vi "Host 25035.vi"() -> ()   [LabVIEW 2018]
uses:
  <instrlib>/niDCPower/nidcpower.llb/niDCPower Measurement Type.ctl
panel:
  in  "2.1_selcur":dbl=0.3 caption="current limit" format="%_6p"
  out "2.1":i32
  out "2.1":bool
  in  "2.0_selcur":dbl=0.3 caption="current limit" format="%_6p"
  out "2.0":i32
  out "2.0":bool
  in  "2.1, V":dbl=5.0 caption="voltage level" format="%_6p"
  in  "2.1_curlim, A":dbl=0.5 caption="current limit" format="%_6p"
  out "2.1_cur, A":dbl caption="measurement" format="%_6g"
  out "2.1 Chart":dbl(graph)=-0.007994936055928669 caption="Waveform Chart 5"
  in  "Период опроса, мс":u32=1
  out "2.0_cur, A":dbl caption="measurement" format="%_6g"
  out "2.0 Chart":dbl(graph)=0.03234747481509968 caption="Waveform Chart 5"
  in  "2.0, V":dbl=5.0 caption="voltage level" format="%_6p"
  in  "2.0_curlim, A":dbl=0.5 caption="current limit" format="%_6p"
  in  "2.0/2.1":refnum<k15>="PXI1Slot4" caption="instrument handle"
  in  "1.1_selcur":dbl=0.3 caption="current limit" format="%_6p"
  out "1.1":i32
  out "1.1":bool
  out "1.1_cur, A":dbl caption="measurement" format="%_6g"
  out "1.1 Chart":dbl(graph)=-0.000235222149982668
  in  "1.1, V":dbl=5.0 caption="voltage level" format="%_6p"
  in  "1.1_curlim, A":dbl=0.5 caption="current limit" format="%_6p"
  in  "Стоп":bool
  in  "Питание":bool
  in  "SEL_T, мс":u32=100
  in  "SIM_SEL":bool
  out "SEL":bool
  in  "0.0_selcur":dbl=0.3 caption="current limit" format="%_6p"
  in  "0.1_selcur":dbl=0.3 caption="current limit" format="%_6p"
  in  "1.0_selcur":dbl=0.3 caption="current limit" format="%_6p"
  out "0.0":i32
  out "0.0":bool
  out "0.1":i32
  out "0.1":bool
  out "1.0":i32
  out "1.0":bool
  in  "0.0, V":dbl=5.0 caption="voltage level" format="%_6p"
  in  "0.0_curlim, A":dbl=0.5 caption="current limit" format="%_6p"
  in  "0.1_curlim, A":dbl=0.5 caption="current limit" format="%_6p"
  out "0.0_cur, A":dbl caption="measurement" format="%_6g"
  out "0.1_cur, A":dbl caption="measurement" format="%_6g"
  in  "0.1, V":dbl=5.0 caption="voltage level" format="%_6p"
  in  "1.0, V":dbl=5.0 caption="voltage level" format="%_6p"
  in  "1.0_curlim, A":dbl=0.5 caption="current limit" format="%_6p"
  out "1.0_cur, A":dbl caption="measurement" format="%_6g"
  out "0.1 Chart":dbl(graph)=-0.0025072983641264367
  out "1.0 Chart":dbl(graph)=-0.0403673797130392
  out "0.0 Chart":dbl(graph)=0.17110122624002952 caption="Waveform Chart 5"
  in  "0.0/0.1":refnum<k15>="PXI1Slot2" caption="instrument handle"
  in  "1.0/1.1":refnum<k15>="PXI1Slot3" caption="instrument handle"
  in  "SEL":path=path "C:/LabView_PRJ/25_035_ИКИ РАН/SEL"
  out "Номер образца":string="0"
  # "Для ТЗЧ:\n0.0 - питание ПЛИС\n1.0 - питание матрицы"
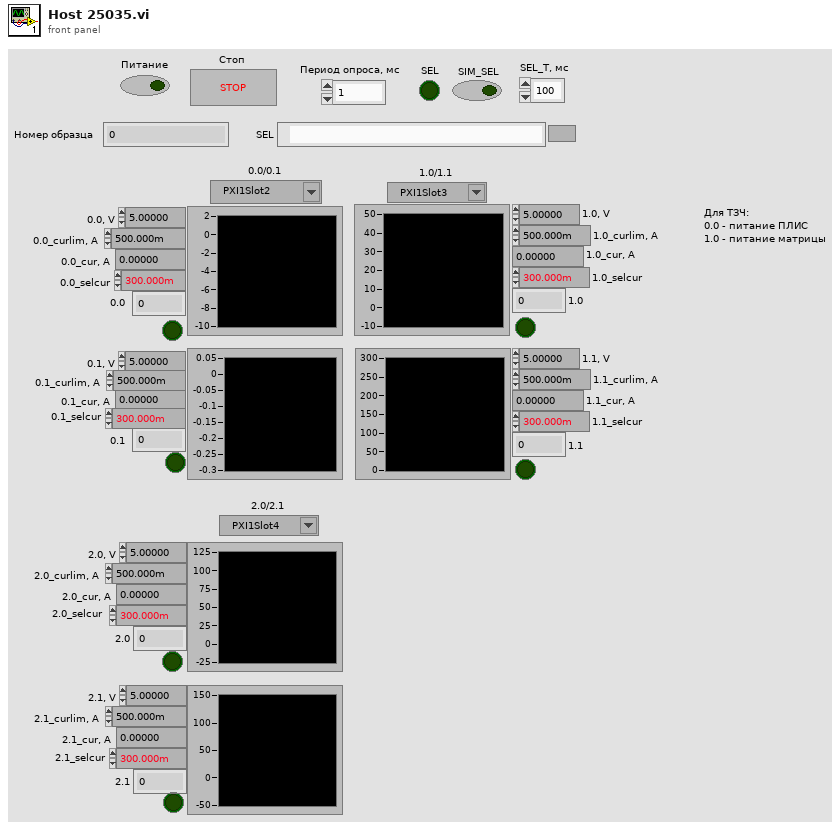
[diagram p1: front panel]
types:
  T1 = enum16{"open", "replace", "create", "open or create", "replace or create", "replace or create with confirmation"}
  T2 = typedef "niDCPower Measurement Type.ctl" = i32
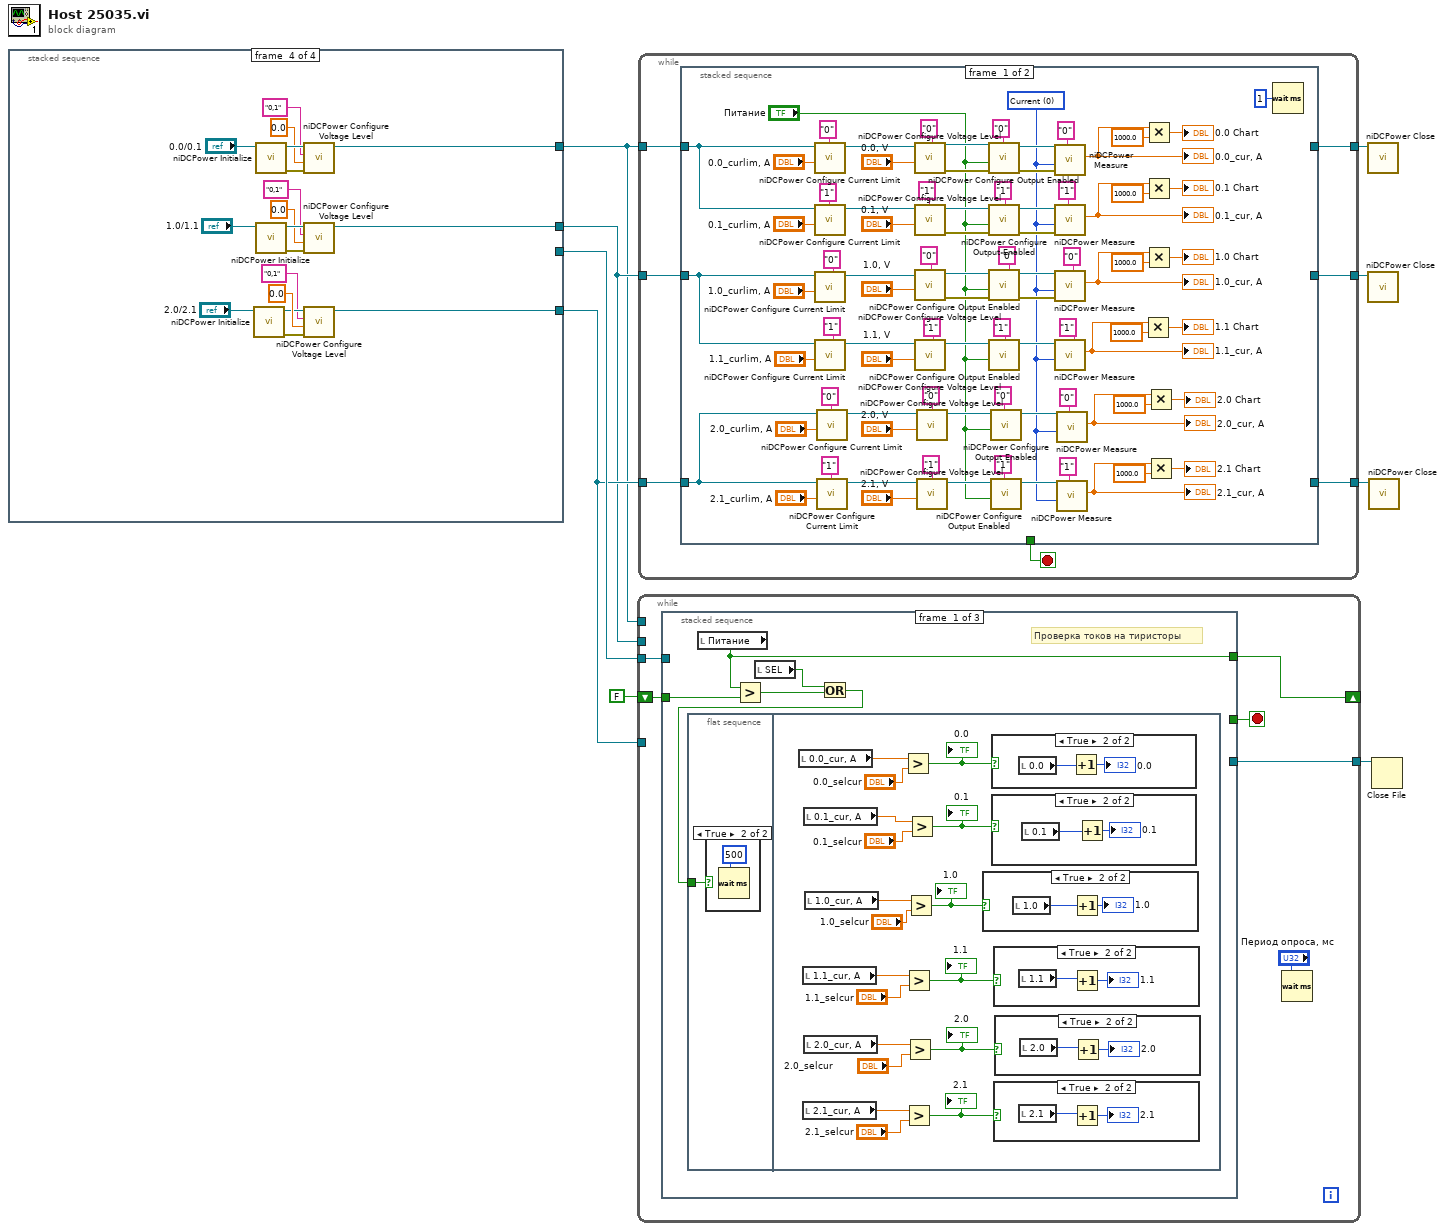
[diagram p0: block diagram]
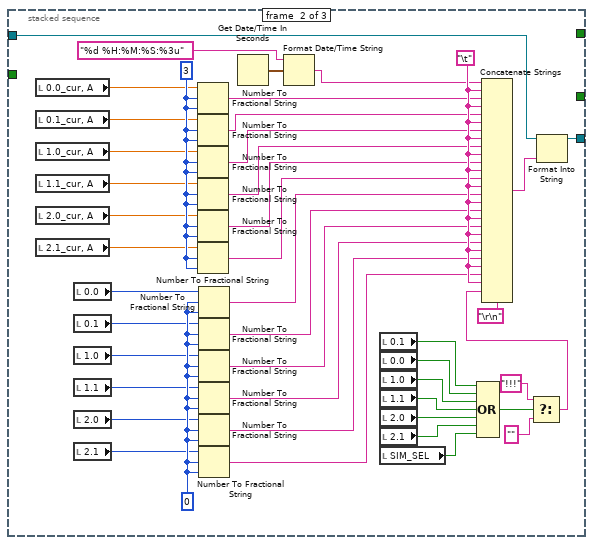
[diagram p9: hidden frame]
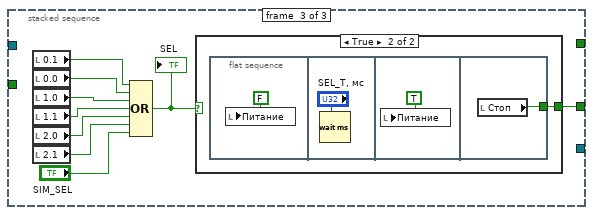
[diagram p10: hidden frame]
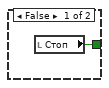
[diagram p11: hidden frame]
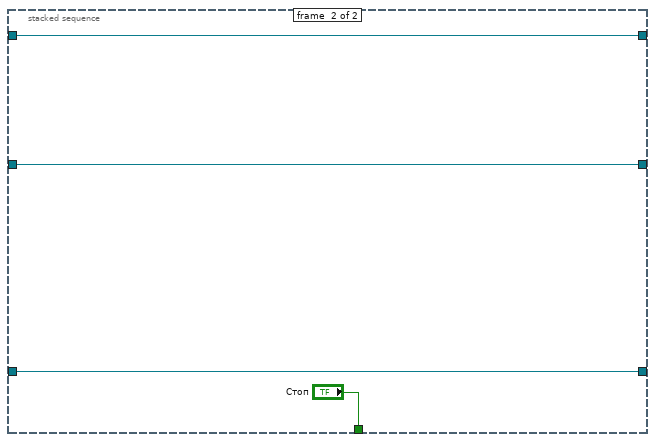
[diagram p12: hidden frame]
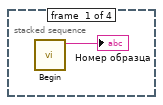
[diagram p13: hidden frame]
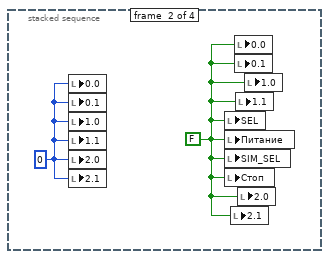
[diagram p14: hidden frame]
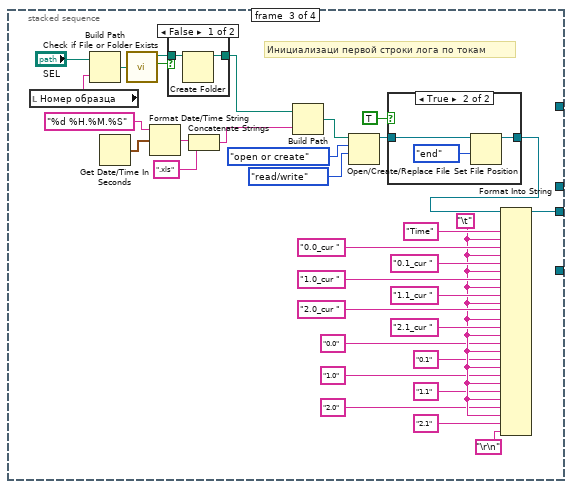
[diagram p15: hidden frame]
diagram:
  n1 = stacked-sequence {
    tunnel: [_ _ _ w60] -> w5
    tunnel: [_ _ _ w59] -> w4
    tunnel: [_ _ w29 _] -> w8
    tunnel: [_ _ _ w53] -> w6
    frame #0 {
      n2 = call "Begin.vi"() -> ("Номер образца 2"=→"Номер образца":string)  [unwired: 11 in]
    }
    frame #1 {
      w12 = 0
      w11 = FALSE
      n3 = local write "0.0"(w12) -> ()
      n4 = local write "0.1"(w12) -> ()
      n5 = local write "1.0"(w12) -> ()
      n6 = local write "1.1"(w12) -> ()
      n7 = local write "2.0"(w12) -> ()
      n8 = local write "2.1"(w12) -> ()
      n9 = local write "SEL"(w11) -> ()
      n10 = local write "Питание"(w11) -> ()
      n11 = local write "SIM_SEL"(w11) -> ()
      n12 = local write "Стоп"(w11) -> ()
      n13 = local write "2.1"(w11) -> ()
      n14 = local write "0.0"(w11) -> ()
      n15 = local write "0.1"(w11) -> ()
      n16 = local write "1.1"(w11) -> ()
      n17 = local write "2.0"(w11) -> ()
      n18 = local write "1.0"(w11) -> ()
    }
    frame #2 {
      w20 = "\t"
      # "Инициализаци первой строки лога по токам"
      n19 = local read "Номер образца"() -> (w41:string)
      n20 = Build Path(base path="SEL", name or relative path=w41) -> (appended path=w43:path)
      n21 = Get Date/Time In Seconds() -> (seconds since 1Jan1904=w36:timestamp)
      n22 = call <vilib>:"Check if File or Folder Exists.vi"("path"=w43) -> ("file or folder exists?"=w44:bool, "dup path"=w45:path)  [unwired: 8 in, 1 out]
      n23 = Format Date/Time String(time format string (%c)="%d %H.%M.%S", seconds (now)=w36) -> (date/time string=w33:string)  [unwired: 1 in]
      n24 = case shown="False" w44 {
        tunnel: w45 -> [w51 w52]
        tunnel: [w50 w52] -> w28
        frame False {
          n25 = Create Folder(path (use dialog)=w51) -> (created path=w50:path)  [unwired: 2 in, 2 out]
        }
        frame True {
        }
      }
      n26 = Concatenate Strings(w33, ".xls" ("string")) -> (w31:string)
      n27 = Build Path(base path=w28, name or relative path=w31) -> (appended path=w34:path)
      n28 = Open/Create/Replace File(file path (use dialog)=w34, operation (0:open)=T1."open or create", access (0:read/write)=enum16{"read/write", "read-only", "write-only"}."read/write") -> (refnum out=w37:refnum<file>)  [unwired: 3 in, 2 out]
      n29 = case shown="True" TRUE {
        tunnel: w37 -> [w46 w49]
        tunnel: [w46 w47] -> w30
        frame False {
        }
        frame True {
          n30 = Set File Position(refnum=w49, from (0:start)=enum16{"start", "end", "current"}."end") -> (refnum out=w47:refnum<file>)  [unwired: 2 in, 1 out]
        }
      }
      n31 = Format Into String(initial string=w30, "Time" ("input 1"), w20, "0.0_cur " ("input 1"), w20, "0.1_cur " ("input 1"), w20, "1.0_cur " ("input 1"), w20, "1.1_cur " ("input 1"), w20, "2.0_cur " ("input 1"), w20, "2.1_cur " ("input 1"), w20, "0.0" ("input 1"), w20, "0.1" ("input 1"), w20, "1.0" ("input 1"), w20, "1.1" ("input 1"), w20, "2.0" ("input 1"), w20, "2.1" ("input 1"), "\r\n") -> (resulting string=w29:refnum<file>)  [unwired: 2 in, 1 out]
    }
    frame #3 {
      n32 = call <instrlib>:"niDCPower Initialize.vi"("resource name"="2.0/2.1") -> ("error out"=w56:errorcluster, "instrument handle out"=w55:refnum<k15>)  [unwired: 3 in, 6 out]
      n33 = call <instrlib>:"niDCPower Initialize.vi"("resource name"="0.0/0.1") -> ("error out"=w67:errorcluster, "instrument handle out"=w69:refnum<k15>)  [unwired: 3 in, 6 out]
      n34 = call <instrlib>:"niDCPower Initialize.vi"("resource name"="1.0/1.1") -> ("error out"=w68:errorcluster, "instrument handle out"=w70:refnum<k15>)  [unwired: 3 in, 6 out]
      n35 = call <instrlib>:"niDCPower Configure Voltage Level.vi"("error in (no error)"=w67, "voltage level"=0.0, "channel name"="0,1", "instrument handle"=w69) -> ("instrument handle out"=w59:refnum<k15>)  [unwired: 6 in, 1 out]
      n36 = call <instrlib>:"niDCPower Configure Voltage Level.vi"("error in (no error)"=w68, "voltage level"=0.0, "channel name"="0,1", "instrument handle"=w70) -> ("instrument handle out"=w60:refnum<k15>)  [unwired: 6 in, 1 out]
      n37 = call <instrlib>:"niDCPower Configure Voltage Level.vi"("error in (no error)"=w56, "voltage level"=0.0, "channel name"="0,1", "instrument handle"=w55) -> ("instrument handle out"=w53:refnum<k15>)  [unwired: 6 in, 1 out]
    }
  }
  n38 = while {
    shift-right: [w76] -> _
    shift-left: FALSE -> [w75]
    tunnel: w8 -> [w74]
    tunnel: [w72] -> w7
    tunnel: w6 -> [_]
    tunnel: w5 -> [_]
    tunnel: w4 -> [_]
    stop <- w73 stop-if-true
    n39 = stacked-sequence {
      tunnel: [w80 _ _] -> w76
      tunnel: w75 -> [w81 _ _]
      tunnel: w74 -> [_ w153 _]
      tunnel: [_ _ w167] -> w73
      tunnel: [_ w152 _] -> w72
      frame #0 {
        # "Проверка токов на тиристоры"
        n40 = flat-sequence {
          tunnel: w77 -> [w82]
          frame #0 {
            n41 = case shown="True" w82 {
              frame False {
              }
              frame True {
                n42 = Wait (ms)(milliseconds to wait=u32 500) -> ()  [unwired: 1 out]
              }
            }
          }
          frame #1 {
            n43 = local read "0.0_cur, A"() -> (w95:dbl)
            n44 = local read "1.1_cur, A"() -> (w92:dbl)
            n45 = local read "2.1_cur, A"() -> (w86:dbl)
            n46 = local read "0.1_cur, A"() -> (w94:dbl)
            n47 = local read "2.0_cur, A"() -> (w87:dbl)
            n48 = local read "1.0_cur, A"() -> (w93:dbl)
            n49 = Greater?(x=w95, y="0.0_selcur") -> (0:w100:bool)
            "0.0" <- w100
            n50 = Greater?(x=w92, y="1.1_selcur") -> (0:w91:bool)
            "1.1" <- w91
            n51 = Greater?(x=w86, y="2.1_selcur") -> (0:w85:bool)
            "2.1" <- w85
            n52 = Greater?(x=w87, y="2.0_selcur") -> (0:w88:bool)
            "2.0" <- w88
            n53 = Greater?(x=w93, y="1.0_selcur") -> (0:w96:bool)
            "1.0" <- w96
            n54 = Greater?(x=w94, y="0.1_selcur") -> (0:w98:bool)
            "0.1" <- w98
            n55 = case shown="True" w96 {
              frame False {
              }
              frame True {
                n56 = local read "1.0"() -> (w109:i32)
                n57 = Increment(x=w109) -> (x+1=→"1.0":i32)
              }
            }
            n58 = case shown="True" w100 {
              frame False {
              }
              frame True {
                n59 = local read "0.0"() -> (w113:i32)
                n60 = Increment(x=w113) -> (x+1=→"0.0":i32)
              }
            }
            n61 = case shown="True" w98 {
              frame False {
              }
              frame True {
                n62 = local read "0.1"() -> (w110:i32)
                n63 = Increment(x=w110) -> (x+1=→"0.1":i32)
              }
            }
            n64 = case shown="True" w91 {
              frame False {
              }
              frame True {
                n65 = local read "1.1"() -> (w107:i32)
                n66 = Increment(x=w107) -> (x+1=→"1.1":i32)
              }
            }
            n67 = case shown="True" w85 {
              frame False {
              }
              frame True {
                n68 = local read "2.1"() -> (w103:i32)
                n69 = Increment(x=w103) -> (x+1=→"2.1":i32)
              }
            }
            n70 = case shown="True" w88 {
              frame False {
              }
              frame True {
                n71 = local read "2.0"() -> (w105:i32)
                n72 = Increment(x=w105) -> (x+1=→"2.0":i32)
              }
            }
          }
        }
        n73 = local read "Питание"() -> (w80:bool)
        n74 = Greater?(x=w80, y=w81) -> (0:w79:bool)
        n75 = local read "SEL"() -> (w78:bool)
        n76 = Or(x=w78, y=w79) -> (x .or. y?=w77:bool)
      }
      frame #1 {
        w150 = i16 0 ("width (-)")
        w151 = i16 3 ("width (-)")
        w149 = "\t"
        n77 = local read "0.0_cur, A"() -> (w148:dbl)
        n78 = local read "0.1_cur, A"() -> (w147:dbl)
        n79 = local read "1.0_cur, A"() -> (w146:dbl)
        n80 = local read "1.1_cur, A"() -> (w145:dbl)
        n81 = local read "2.0_cur, A"() -> (w144:dbl)
        n82 = local read "2.1_cur, A"() -> (w143:dbl)
        n83 = local read "0.0"() -> (w142:i32)
        n84 = local read "0.1"() -> (w141:i32)
        n85 = local read "1.0"() -> (w140:i32)
        n86 = local read "1.1"() -> (w139:i32)
        n87 = local read "2.0"() -> (w138:i32)
        n88 = local read "2.1"() -> (w137:i32)
        n89 = Number To Fractional String(number=w148, width (-)=w151, precision (6)=w151) -> (F-format string=w135:string)  [unwired: 1 in]
        n90 = Number To Fractional String(number=w147, width (-)=w151, precision (6)=w151) -> (F-format string=w134:string)  [unwired: 1 in]
        n91 = Number To Fractional String(number=w146, width (-)=w151, precision (6)=w151) -> (F-format string=w133:string)  [unwired: 1 in]
        n92 = Number To Fractional String(number=w145, width (-)=w151, precision (6)=w151) -> (F-format string=w132:string)  [unwired: 1 in]
        n93 = Number To Fractional String(number=w144, width (-)=w151, precision (6)=w151) -> (F-format string=w131:string)  [unwired: 1 in]
        n94 = Number To Fractional String(number=w143, width (-)=w151, precision (6)=w151) -> (F-format string=w130:string)  [unwired: 1 in]
        n95 = Number To Fractional String(number=w142, width (-)=w150, precision (6)=w150) -> (F-format string=w129:string)  [unwired: 1 in]
        n96 = Number To Fractional String(number=w141, width (-)=w150, precision (6)=w150) -> (F-format string=w128:string)  [unwired: 1 in]
        n97 = Number To Fractional String(number=w140, width (-)=w150, precision (6)=w150) -> (F-format string=w127:string)  [unwired: 1 in]
        n98 = Number To Fractional String(number=w139, width (-)=w150, precision (6)=w150) -> (F-format string=w126:string)  [unwired: 1 in]
        n99 = Number To Fractional String(number=w138, width (-)=w150, precision (6)=w150) -> (F-format string=w125:string)  [unwired: 1 in]
        n100 = Number To Fractional String(number=w137, width (-)=w150, precision (6)=w150) -> (F-format string=w124:string)  [unwired: 1 in]
        n101 = Get Date/Time In Seconds() -> (seconds since 1Jan1904=w158:timestamp)
        n102 = Format Date/Time String(time format string (%c)="%d %H:%M:%S:%3u", seconds (now)=w158) -> (date/time string=w136:string)  [unwired: 1 in]
        n103 = local read "0.1"() -> (w121:bool)
        n104 = local read "0.0"() -> (w120:bool)
        n105 = local read "1.0"() -> (w119:bool)
        n106 = local read "1.1"() -> (w118:bool)
        n107 = local read "2.0"() -> (w117:bool)
        n108 = local read "2.1"() -> (w116:bool)
        n109 = local read "SIM_SEL"() -> (w115:bool)
        n110 = Compound Arithmetic op=OR(w121, w120, w119, w118, w117, w116, w115) -> (w114:bool)
        n111 = Select(t="!!!", s=w114, f="") -> (s? t:f=w123:string)
        n112 = Concatenate Strings(w136, w149, w135, w149, w134, w149, w133, w149, w132, w149, w131, w149, w130, w149, w129, w149, w128, w149, w127, w149, w126, w149, w125, w149, w124, w149, w123, "\r\n") -> (w157:string)
        n113 = Format Into String(initial string=w153, w157) -> (resulting string=w152:refnum<file>)  [unwired: 2 in, 1 out]
      }
      frame #2 {
        n114 = local read "0.1"() -> (w166:bool)
        n115 = local read "0.0"() -> (w164:bool)
        n116 = local read "1.0"() -> (w163:bool)
        n117 = local read "1.1"() -> (w162:bool)
        n118 = local read "2.0"() -> (w161:bool)
        n119 = local read "2.1"() -> (w160:bool)
        n120 = Compound Arithmetic op=OR(w166, w164, w163, w162, w161, w160, "SIM_SEL") -> (w165:bool)
        "SEL" <- w165
        n121 = case shown="True" w165 {
          tunnel: [w168 w169] -> w167
          frame False {
            n122 = local read "Стоп"() -> (w168:bool)
          }
          frame True {
            n123 = flat-sequence {
              tunnel: [w173] -> w169
              frame #0 {
                n124 = local write "Питание"(FALSE ("SYS_RESET")) -> ()
              }
              frame #1 {
                n125 = Wait (ms)(milliseconds to wait="SEL_T, мс") -> ()  [unwired: 1 out]
              }
              frame #2 {
                n126 = local write "Питание"(TRUE ("SYS_RESET")) -> ()
              }
              frame #3 {
                n127 = local read "Стоп"() -> (w173:bool)
              }
            }
          }
        }
      }
    }
    n128 = Wait (ms)(milliseconds to wait="Период опроса, мс") -> ()  [unwired: 1 out]
  }
  n129 = while {
    tunnel: w4 -> [w180]
    tunnel: w6 -> [w178]
    tunnel: w5 -> [w179]
    tunnel: [w177] -> w3
    tunnel: [w176] -> w2
    tunnel: [w175] -> w1
    stop <- w174 stop-if-true
    n130 = stacked-sequence {
      tunnel: w178 -> [w184 w266]
      tunnel: w179 -> [w183 w267]
      tunnel: w180 -> [w182 w268]
      tunnel: [_ w268] -> w177
      tunnel: [_ w267] -> w176
      tunnel: [_ w266] -> w175
      tunnel: [_ "Стоп"] -> w174
      frame #0 {
        w185 = T2 0 items=["Current", "Voltage"] ("measurement type")
        n131 = call <instrlib>:"niDCPower Configure Current Limit.vi"("current limit"="0.0_curlim, A", "channel name"="0", "instrument handle"=w182) -> ("instrument handle out"=w253:refnum<k15>)  [unwired: 7 in, 1 out]
        n132 = call <instrlib>:"niDCPower Configure Current Limit.vi"("current limit"="0.1_curlim, A", "channel name"="1", "instrument handle"=w182) -> ("instrument handle out"=w254:refnum<k15>)  [unwired: 7 in, 1 out]
        n133 = call <instrlib>:"niDCPower Configure Current Limit.vi"("current limit"="1.0_curlim, A", "channel name"="0", "instrument handle"=w183) -> ("instrument handle out"=w236:refnum<k15>)  [unwired: 7 in, 1 out]
        n134 = call <instrlib>:"niDCPower Configure Current Limit.vi"("current limit"="1.1_curlim, A", "channel name"="1", "instrument handle"=w183) -> ("instrument handle out"=w216:refnum<k15>)  [unwired: 7 in, 1 out]
        n135 = call <instrlib>:"niDCPower Configure Current Limit.vi"("current limit"="2.0_curlim, A", "channel name"="0", "instrument handle"=w184) -> ("instrument handle out"=w207:refnum<k15>)  [unwired: 7 in, 1 out]
        n136 = call <instrlib>:"niDCPower Configure Current Limit.vi"("current limit"="2.1_curlim, A", "channel name"="1", "instrument handle"=w184) -> ("instrument handle out"=w188:refnum<k15>)  [unwired: 7 in, 1 out]
        n137 = call <instrlib>:"niDCPower Configure Voltage Level.vi"("voltage level"="0.0, V", "channel name"="0", "instrument handle"=w253) -> ("error out"=w246:errorcluster, "instrument handle out"=w249:refnum<k15>)  [unwired: 7 in]
        n138 = call <instrlib>:"niDCPower Configure Voltage Level.vi"("voltage level"="0.1, V", "channel name"="1", "instrument handle"=w254) -> ("error out"=w247:errorcluster, "instrument handle out"=w248:refnum<k15>)  [unwired: 7 in]
        n139 = call <instrlib>:"niDCPower Configure Voltage Level.vi"("voltage level"="1.0, V", "channel name"="0", "instrument handle"=w236) -> ("error out"=w240:errorcluster, "instrument handle out"=w241:refnum<k15>)  [unwired: 7 in]
        n140 = call <instrlib>:"niDCPower Configure Voltage Level.vi"("voltage level"="1.1, V", "channel name"="1", "instrument handle"=w216) -> ("instrument handle out"=w214:refnum<k15>)  [unwired: 7 in, 1 out]
        n141 = call <instrlib>:"niDCPower Configure Voltage Level.vi"("voltage level"="2.0, V", "channel name"="0", "instrument handle"=w207) -> ("instrument handle out"=w206:refnum<k15>)  [unwired: 7 in, 1 out]
        n142 = call <instrlib>:"niDCPower Configure Voltage Level.vi"("voltage level"="2.1, V", "channel name"="1", "instrument handle"=w188) -> ("instrument handle out"=w189:refnum<k15>)  [unwired: 7 in, 1 out]
        n143 = call <instrlib>:"niDCPower Configure Output Enabled.vi"("error in (no error)"=w246, "output enabled"="Питание", "channel name"="0", "instrument handle"=w249) -> ("error out"=w258:errorcluster, "instrument handle out"=w257:refnum<k15>)  [unwired: 6 in]
        n144 = call <instrlib>:"niDCPower Configure Output Enabled.vi"("error in (no error)"=w247, "output enabled"="Питание", "channel name"="1", "instrument handle"=w248) -> ("error out"=w259:errorcluster, "instrument handle out"=w260:refnum<k15>)  [unwired: 6 in]
        n145 = call <instrlib>:"niDCPower Configure Output Enabled.vi"("error in (no error)"=w240, "output enabled"="Питание", "channel name"="0", "instrument handle"=w241) -> ("error out"=w232:errorcluster, "instrument handle out"=w233:refnum<k15>)  [unwired: 6 in]
        n146 = call <instrlib>:"niDCPower Configure Output Enabled.vi"("output enabled"="Питание", "channel name"="1", "instrument handle"=w214) -> ("instrument handle out"=w212:refnum<k15>)  [unwired: 7 in, 1 out]
        n147 = call <instrlib>:"niDCPower Configure Output Enabled.vi"("output enabled"="Питание", "channel name"="0", "instrument handle"=w206) -> ("instrument handle out"=w205:refnum<k15>)  [unwired: 7 in, 1 out]
        n148 = call <instrlib>:"niDCPower Configure Output Enabled.vi"("output enabled"="Питание", "channel name"="1", "instrument handle"=w189) -> ("instrument handle out"=w190:refnum<k15>)  [unwired: 7 in, 1 out]
        n149 = call <instrlib>:"niDCPower Measure.vi"("error in (no error)"=w258, "measurement type"=w185, "channel name"="0", "instrument handle"=w257) -> ("measurement"=w225:dbl)  [unwired: 5 in, 2 out]
        "0.0_cur, A" <- w225
        n150 = call <instrlib>:"niDCPower Measure.vi"("error in (no error)"=w259, "measurement type"=w185, "channel name"="1", "instrument handle"=w260) -> ("measurement"=w228:dbl)  [unwired: 5 in, 2 out]
        "0.1_cur, A" <- w228
        n151 = call <instrlib>:"niDCPower Measure.vi"("error in (no error)"=w232, "measurement type"=w185, "channel name"="0", "instrument handle"=w233) -> ("measurement"=w226:dbl)  [unwired: 5 in, 2 out]
        "1.0_cur, A" <- w226
        n152 = call <instrlib>:"niDCPower Measure.vi"("measurement type"=w185, "channel name"="1", "instrument handle"=w212) -> ("measurement"=w210:dbl)  [unwired: 6 in, 2 out]
        "1.1_cur, A" <- w210
        n153 = call <instrlib>:"niDCPower Measure.vi"("measurement type"=w185, "channel name"="0", "instrument handle"=w205) -> ("measurement"=w204:dbl)  [unwired: 6 in, 2 out]
        "2.0_cur, A" <- w204
        n154 = call <instrlib>:"niDCPower Measure.vi"("measurement type"=w185, "channel name"="1", "instrument handle"=w190) -> ("measurement"=w191:dbl)  [unwired: 6 in, 2 out]
        "2.1_cur, A" <- w191
        n155 = Multiply(x=w210, y=1000.0) -> (x*y=→"1.1 Chart":dbl)
        n156 = Multiply(x=w225, y=1000.0) -> (x*y=→"0.0 Chart":dbl)
        n157 = Multiply(x=w228, y=1000.0) -> (x*y=→"0.1 Chart":dbl)
        n158 = Multiply(x=w226, y=1000.0) -> (x*y=→"1.0 Chart":dbl)
        n159 = Multiply(x=w204, y=1000.0) -> (x*y=→"2.0 Chart":dbl)
        n160 = Multiply(x=w191, y=1000.0) -> (x*y=→"2.1 Chart":dbl)
        n161 = Wait (ms)(milliseconds to wait=u32 1) -> ()  [unwired: 1 out]
      }
      frame #1 {
      }
    }
  }
  n162 = call <instrlib>:"niDCPower Close.vi"("instrument handle"=w3) -> ()  [unwired: 10 in, 1 out]
  n163 = call <instrlib>:"niDCPower Close.vi"("instrument handle"=w2) -> ()  [unwired: 10 in, 1 out]
  n164 = call <instrlib>:"niDCPower Close.vi"("instrument handle"=w1) -> ()  [unwired: 10 in, 1 out]
  n165 = Close File(refnum=w7) -> ()  [unwired: 1 in, 2 out]
